vi "Format String to Number.vi"() -> ()   [LabVIEW 2011]
panel:
  in  "String":string="0.123456789"
  out "value":dbl format="%#_8g"
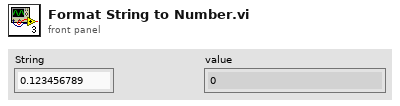
[diagram p1: front panel]
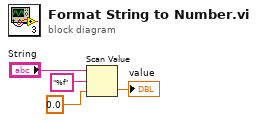
[diagram p0: block diagram]
diagram:
  n1 = Scan Value(string="String", format string="%f", default (0 dbl)=0.0) -> (value=→"value":dbl)  [unwired: 1 out]
